vi "Indefinite Integral of Polynomial (DBL).vi"(11 "P(x)":dbl[](array[numeric])) -> (0 "error":i32, 3 "Indefinite Integral of P(x)":dbl[](array[numeric]))   [LabVIEW 2017, in "NI_AALPro.lvlib"]
doc: "Calculates the indefinite integral of <B>P(x)</B>. Wire data to the <B>P(x)</B> input to determine the polymorphic instance to use or manually select the instance."
uses:
  NI_AALPro.lvlib
  Ramp Pattern by Samples.vi
  NI_AALBase.lvlib
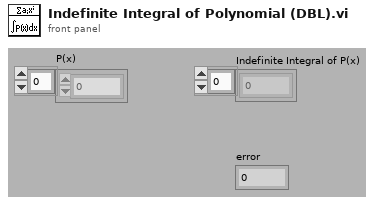
[diagram p1: front panel]
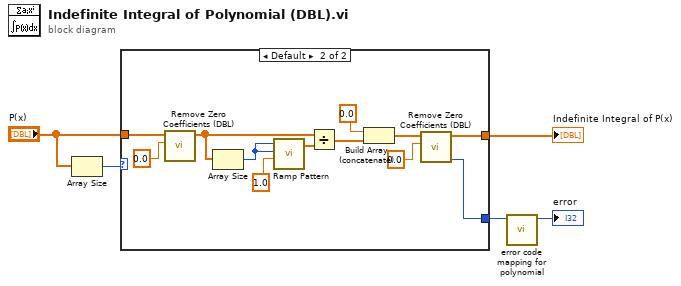
[diagram p0: block diagram]
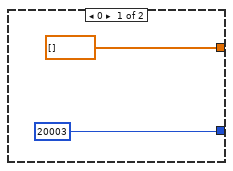
[diagram p2: hidden frame]
diagram:
  n1 = Array Size(array="P(x)") -> (size(s)=w4:i32)
  n2 = case shown="Default" w4 {
    tunnel: [dbl[] [] ("BDL") w14] -> w3
    tunnel: "P(x)" -> [_ w18]
    tunnel: [20003 ("empty array") w13] -> w2
    frame 0 {
    }
    frame Default {
      n3 = call "Remove Zero Coefficients (DBL).vi"("threshold"=0.0, "P(x) In"=w18) -> ("P(x) Out"=w9:dbl[])  [unwired: 7 in, 2 out]
      n4 = Array Size(array=w9) -> (size(s)=w12:i32)
      n5 = call-poly "Ramp Pattern.vi"("start"=1.0, "end"=w12, "samples"=w12) -> ("Ramp Pattern"=w8:dbl[])  [unwired: 7 in, 1 out]
      n6 = Divide(x=w9, y=w8) -> (x/y=w10:dbl[])
      n7 = Build Array (concatenate)(0.0, w10) -> (w15:dbl[])
      n8 = call "Remove Zero Coefficients (DBL).vi"("threshold"=0.0, "P(x) In"=w15) -> ("error"=w13:i32, "P(x) Out"=w14:dbl[])  [unwired: 7 in, 1 out]
    }
  }
  "Indefinite Integral of P(x)" <- w3
  n9 = call "error code mapping for polynomial.vi"("error in"=w2) -> ("error out"=→"error":i32)  [unwired: 10 in]
